vi "SaveLoadPreview-main.vi"(6 "error in":errorcluster, 10 "Prev-Save-Load":T1) -> (4 "error out 3":errorcluster)   [LabVIEW 2016, in "SaveLoad.lvlib"]
doc: "Takes a vi and saves or loads set values depending on which cluster value is chosen"
uses:
  SaveLoad.lvlib
  saveloadprev.ctl
  Beam Line Sections/R45.vi
  Beam Line Sections/LowEnd.vi
  Beam Line Sections/Source A.vi
  Tools/Scale.vi
  Tools/injector magnet.vi
  High energy end/High energy llb.lvlib
  controls/beamline sections.lvlib
  R30/R30  library.lvlib
  Transmission/transmission.lvlib
  low energy end/Low energy end/Low energy end llb.lvlib
  Features/features/features.lvlib
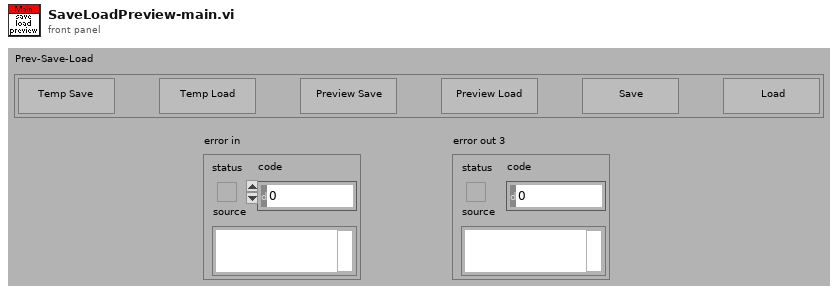
[diagram p1: front panel]
types:
  T1 = typedef "saveloadprev.ctl" = cluster{"Temp Save":bool, "Temp Load":bool, "Save":bool, "Load":bool, "Preview Save":bool, "Preview Load":bool}
  T2 = enum16{"open", "replace", "create", "open or create", "replace or create", "replace or create with confirmation"}
  T3 = typedef "prev-save-load-enum.ctl" = enum16{"Temp Save", "Temp Load", "Save", "Load", "Preview Save", "Preview Load"}
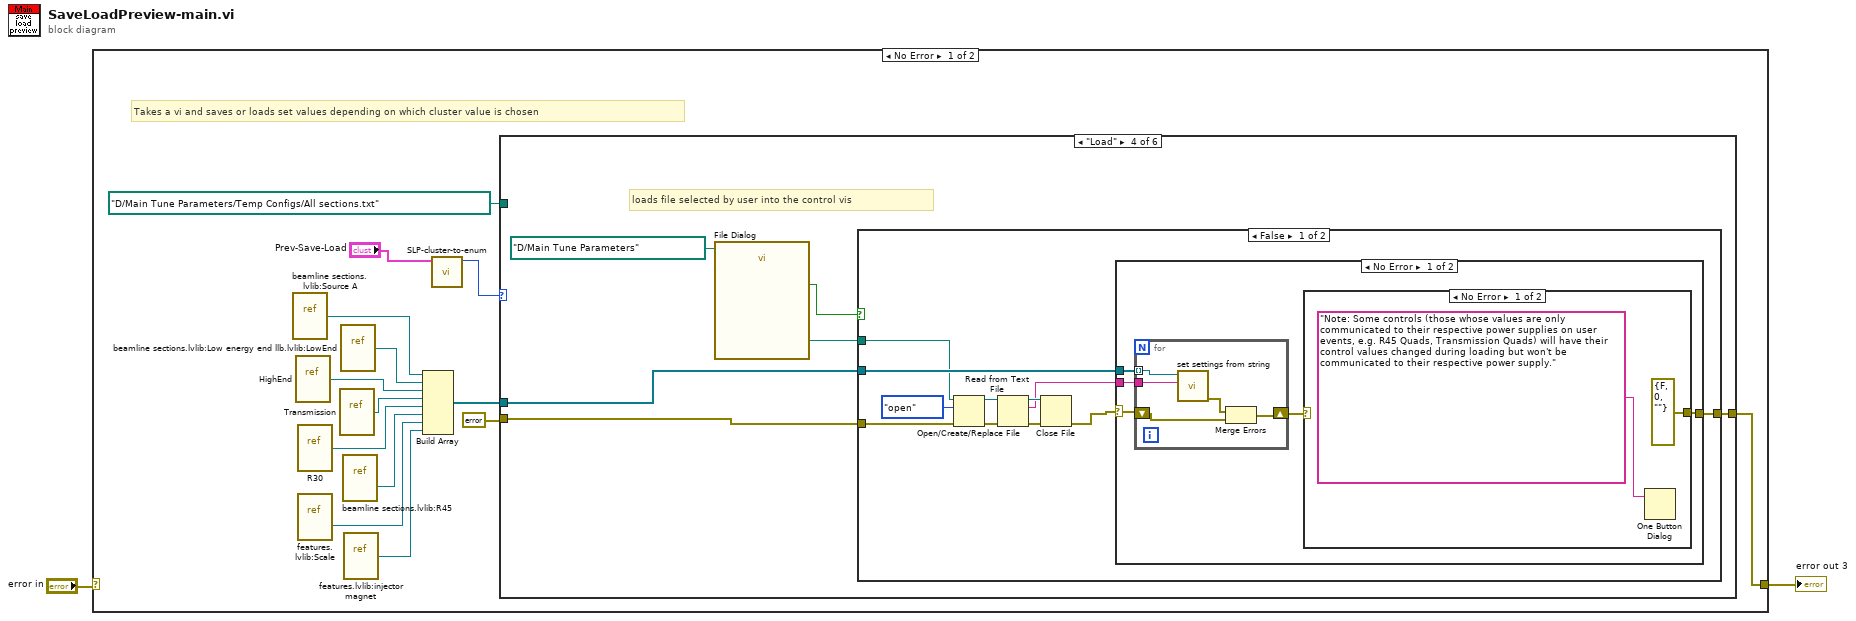
[diagram p0: block diagram]
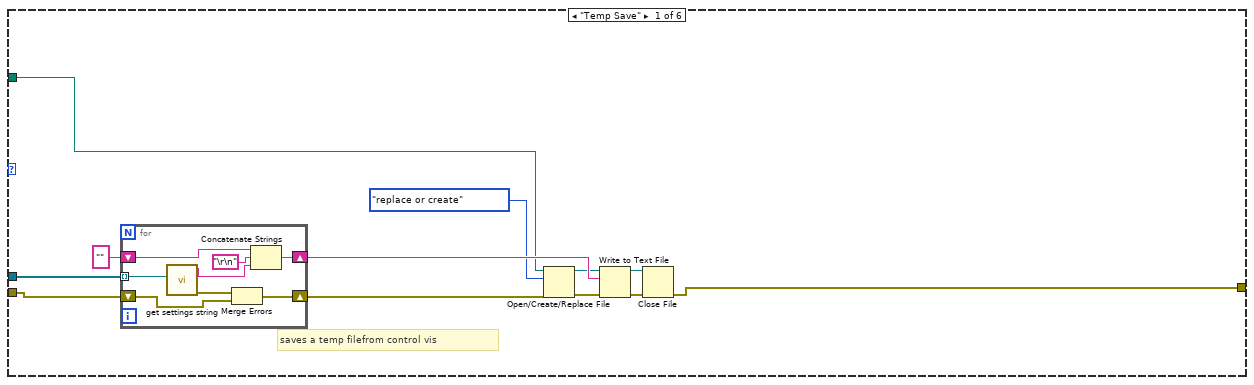
[diagram p2: hidden frame]
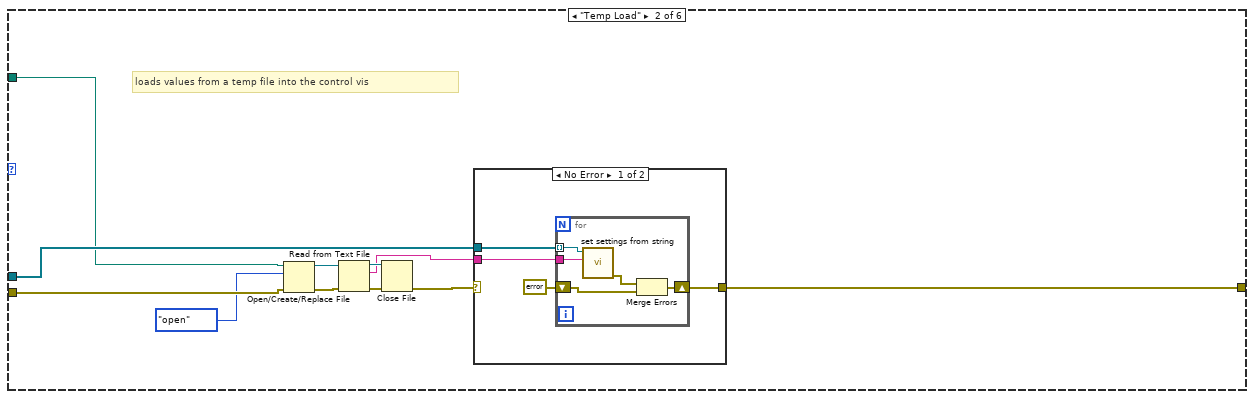
[diagram p3: hidden frame]
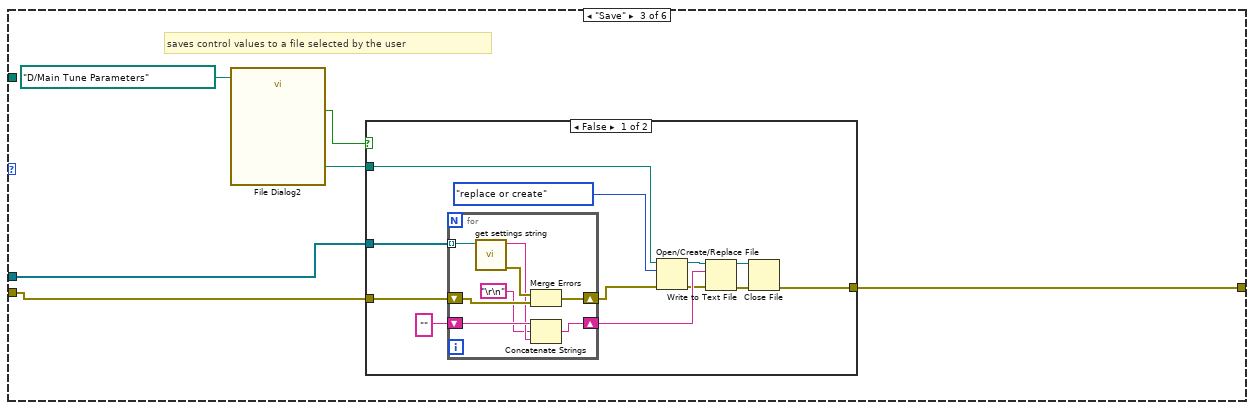
[diagram p5: hidden frame]
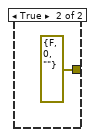
[diagram p6: hidden frame]
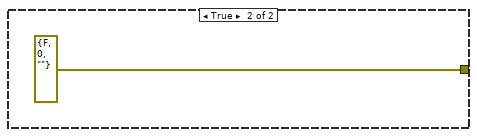
[diagram p9: hidden frame]
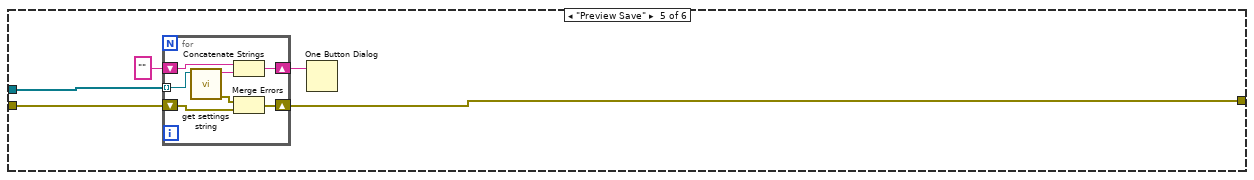
[diagram p10: hidden frame]
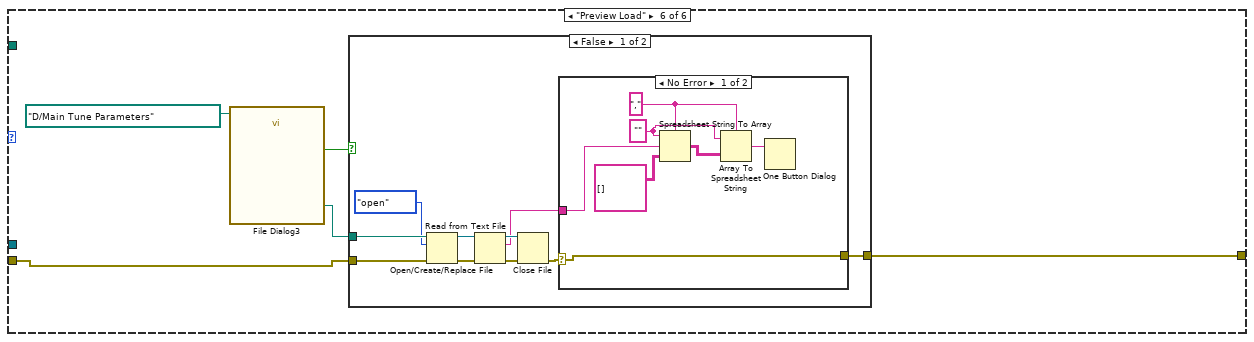
[diagram p11: hidden frame]
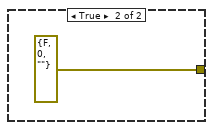
[diagram p13: hidden frame]
diagram:
  n1 = case shown="No Error" "error in" {
    selector: "error in" -> [_ w153]
    tunnel: [w16 w153] -> w2
    frame No Error {
      # "Takes a vi and saves or loads set values depending on which cluster value is chosen"
      n2 = vi-ref "beamline sections.lvlib:Source A.vi"() -> (w10:refnum<vi>)
      n3 = vi-ref "HighEnd.vi"() -> (w14:refnum<vi>)
      n4 = vi-ref "R30.vi"() -> (w13:refnum<vi>)
      n5 = vi-ref "features.lvlib:Scale.vi"() -> (w9:refnum<vi>)
      n6 = vi-ref "Transmission.vi"() -> (w15:refnum<vi>)
      n7 = vi-ref "beamline sections.lvlib:Low energy end llb.lvlib:LowEnd.vi"() -> (w11:refnum<vi>)
      n8 = vi-ref "beamline sections.lvlib:R45.vi"() -> (w12:refnum<vi>)
      n9 = vi-ref "features.lvlib:injector magnet.vi"() -> (w8:refnum<vi>)
      n10 = Build Array(w10, w11, w14, w15, w13, w12, w9, w8) -> (w7:refnum<vi>[])
      n11 = call "SLP-cluster-to-enum.vi"("Prev-Save-Load"="Prev-Save-Load") -> ("Prev-Save-Load enum"=w5:T3)  [unwired: 10 in]
      n12 = case shown="\"Load\"" w5 {
        tunnel: errorcluster {"status"=FALSE, "code"=0, "source"=""} ("error IO") -> [w17 w39 w62 w88 w117 w130]
        tunnel: [w24 w43 w61 w89 w118 w133] -> w16
        tunnel: w7 -> [w22 w45 w63 w90 w121 _]
        tunnel: path "D:/Main Tune Parameters/Temp Configs/All sections.txt" ("file path (use dialog)") -> [w20 w40 _ _ _ _]
        frame "Temp Save" {
          # "saves a temp filefrom control vis"
          n13 = for {
            shift-right: [w35] -> w28
            shift-left: "" -> [w34]
            tunnel: w22 -> [w33] mode=indexing
            shift-right: [w30] -> w23
            shift-left: w17 -> [w29]
            n14 = call "get settings string.vi"("VI in"=w33) -> ("error out"=w32:errorcluster, "Settings string"=w31:string)  [unwired: 9 in]
            n15 = Merge Errors(w32, w29) -> (w30:errorcluster)
            n16 = Concatenate Strings(w34, "\r\n", w31) -> (w35:string)
          }
          n17 = Open/Create/Replace File(file path (use dialog)=w20, error in=w23, operation (0:open)=T2."replace or create") -> (refnum out=w19:refnum<file>, error out=w21:errorcluster)  [unwired: 3 in, 1 out]
          n18 = Write to Text File(file (use dialog)=w19, text=w28, error in=w21) -> (refnum out=w26:refnum<file>, error out=w25:errorcluster)  [unwired: 1 in, 1 out]
          n19 = Close File(refnum=w26, error in=w25) -> (error out=w24:errorcluster)  [unwired: 1 out]
        }
        frame "Temp Load" {
          # "loads values from a temp file into the control vis"
          n20 = Open/Create/Replace File(file path (use dialog)=w40, error in=w39, operation (0:open)=T2."open") -> (refnum out=w41:refnum<file>, error out=w42:errorcluster)  [unwired: 3 in, 1 out]
          n21 = Read from Text File(file (use dialog)=w41, error in=w42) -> (refnum out=w47:refnum<file>, text=w44:string, error out=w46:errorcluster)  [unwired: 3 out]
          n22 = Close File(refnum=w47, error in=w46) -> (error out=w37:errorcluster)  [unwired: 1 out]
          n23 = case shown="No Error" w37 {
            selector: w37 -> [_ w57]
            tunnel: w45 -> [w51 _]
            tunnel: w44 -> [w50 _]
            tunnel: [w49 w57] -> w43
            frame No Error {
              n24 = for {
                tunnel: w51 -> [w55] mode=indexing
                tunnel: w50 -> [w56]
                shift-right: [w54] -> w49
                shift-left: errorcluster {"status"=FALSE, "code"=0, "source"=""} ("error IO") -> [w52]
                n25 = call "set settings from string.vi"("String"=w56, "VI in"=w55) -> ("error out"=w53:errorcluster)  [unwired: 9 in]
                n26 = Merge Errors(w53, w52) -> (w54:errorcluster)
              }
            }
            frame Error {
            }
          }
        }
        frame "Save" {
          # "saves control values to a file selected by the user"
          n27 = call "File Dialog2"("start path"=path "D:/Main Tune Parameters") -> ("selected path"=w59:path, "cancelled"=w58:bool)  [unwired: 11 in, 2 out]
          n28 = case shown="False" w58 {
            tunnel: w63 -> [w72 _]
            tunnel: w62 -> [w71 _]
            tunnel: [w64 errorcluster {"status"=FALSE, "code"=0, "source"=""} ("error out")] -> w61
            tunnel: w59 -> [w65 _]
            frame False {
              n29 = for {
                tunnel: w72 -> [w83] mode=indexing
                shift-right: [w81] -> w66
                shift-left: w71 -> [w80]
                shift-right: [w79] -> w70
                shift-left: "" -> [w78]
                n30 = call "get settings string.vi"("VI in"=w83) -> ("error out"=w82:errorcluster, "Settings string"=w77:string)  [unwired: 9 in]
                n31 = Merge Errors(w82, w80) -> (w81:errorcluster)
                n32 = Concatenate Strings(w78, "\r\n", w77) -> (w79:string)
              }
              n33 = Open/Create/Replace File(file path (use dialog)=w65, error in=w66, operation (0:open)=T2."replace or create") -> (refnum out=w68:refnum<file>, error out=w67:errorcluster)  [unwired: 1 in, 3 out]
              n34 = Write to Text File(file (use dialog)=w68, text=w70, error in=w67) -> (refnum out=w75:refnum<file>, error out=w74:errorcluster)  [unwired: 1 in, 1 out]
              n35 = Close File(refnum=w75, error in=w74) -> (error out=w64:errorcluster)  [unwired: 1 out]
            }
            frame True {
            }
          }
        }
        frame "Load" {
          # "loads file selected by user into the control vis"
          n36 = call "File Dialog"("start path"=path "D:/Main Tune Parameters") -> ("selected path"=w87:path, "cancelled"=w85:bool)  [unwired: 11 in, 2 out]
          n37 = case shown="False" w85 {
            tunnel: w90 -> [w99 _]
            tunnel: [w97 errorcluster {"status"=FALSE, "code"=0, "source"=""} ("error out")] -> w89
            tunnel: w88 -> [w96 _]
            tunnel: w87 -> [w92 _]
            frame False {
              n38 = Open/Create/Replace File(file path (use dialog)=w92, error in=w96, operation (0:open)=T2."open") -> (refnum out=w94:refnum<file>, error out=w95:errorcluster)  [unwired: 3 in, 1 out]
              n39 = Read from Text File(file (use dialog)=w94, error in=w95) -> (refnum out=w100:refnum<file>, text=w98:string, error out=w101:errorcluster)  [unwired: 3 out]
              n40 = Close File(refnum=w100, error in=w101) -> (error out=w91:errorcluster)  [unwired: 1 out]
              n41 = case shown="No Error" w91 {
                selector: w91 -> [w104 w115]
                tunnel: w99 -> [w106 _]
                tunnel: w98 -> [w105 _]
                tunnel: [w102 w115] -> w97
                frame No Error {
                  n42 = for {
                    tunnel: w106 -> [w113] mode=indexing
                    tunnel: w105 -> [w114]
                    shift-right: [w112] -> w103
                    shift-left: w104 -> [w110]
                    n43 = call "set settings from string.vi"("String"=w114, "VI in"=w113) -> ("error out"=w111:errorcluster)  [unwired: 9 in]
                    n44 = Merge Errors(w111, w110) -> (w112:errorcluster)
                  }
                  n45 = case shown="No Error" w103 {
                    selector: w103 -> [_ w109]
                    tunnel: [errorcluster {"status"=FALSE, "code"=0, "source"=""} ("error IO") w109] -> w102
                    frame No Error {
                      n46 = One Button Dialog(message="Note: Some controls (those whose values are only communicated to their respective power supplies on user events, e.g. R45 Quads, Transmission Quads) will have their control values changed during loading but won't be communicated to their respective power supply.") -> ()  [unwired: 1 in, 1 out]
                    }
                    frame Error {
                    }
                  }
                }
                frame Error {
                }
              }
            }
            frame True {
            }
          }
        }
        frame "Preview Save" {
          n47 = for {
            tunnel: w121 -> [w128] mode=indexing
            shift-right: [w126] -> w118
            shift-left: w117 -> [w125]
            shift-right: [w123] -> w119
            shift-left: "" -> [w122]
            n48 = call "get settings string.vi"("VI in"=w128) -> ("error out"=w127:errorcluster, "Settings string"=w124:string)  [unwired: 9 in]
            n49 = Concatenate Strings(w122, w124) -> (w123:string)
            n50 = Merge Errors(w127, w125) -> (w126:errorcluster)
          }
          n51 = One Button Dialog(message=w119) -> ()  [unwired: 1 in, 1 out]
        }
        frame "Preview Load" {
          n52 = call "File Dialog3"("start path"=path "D:/Main Tune Parameters") -> ("selected path"=w131:path, "cancelled"=w129:bool)  [unwired: 11 in, 2 out]
          n53 = case shown="False" w129 {
            tunnel: [w134 errorcluster {"status"=FALSE, "code"=0, "source"=""} ("error out")] -> w133
            tunnel: w131 -> [w140 _]
            tunnel: w130 -> [w136 _]
            frame False {
              n54 = Open/Create/Replace File(file path (use dialog)=w140, error in=w136, operation (0:open)=T2."open") -> (refnum out=w137:refnum<file>, error out=w138:errorcluster)  [unwired: 3 in, 1 out]
              n55 = Read from Text File(file (use dialog)=w137, error in=w138) -> (refnum out=w142:refnum<file>, text=w141:string, error out=w143:errorcluster)  [unwired: 3 out]
              n56 = Close File(refnum=w142, error in=w143) -> (error out=w135:errorcluster)  [unwired: 1 out]
              n57 = case shown="No Error" w135 {
                selector: w135 -> [w144 w151]
                tunnel: w141 -> [w149 _]
                tunnel: [w144 w151] -> w134
                frame No Error {
                  w146 = "," ("delimiter (Tab)")
                  w147 = "" ("format string")
                  n58 = Spreadsheet String To Array(delimiter (Tab)=w146, format string=w147, spreadsheet string=w149, array type (2D Dbl)=string[][] []) -> (array=w148:string[][])
                  n59 = Array To Spreadsheet String(delimiter (Tab)=w146, array=w148, 3:w147) -> (spreadsheet string=w145:string)
                  n60 = One Button Dialog(message=w145) -> ()  [unwired: 1 in, 1 out]
                }
                frame Error {
                }
              }
            }
            frame True {
            }
          }
        }
      }
    }
    frame Error {
    }
  }
  "error out 3" <- w2
